vi "KRing Test.vi"() -> ()   [LabVIEW 2015]
uses:
  Controls/KRing/KRing.xctl
panel:
  out "Array":i16[](array[numeric])
  in  "Array":i16[](array[numeric])
  in  "KRing":i16(xcontrol)
  in  "Apply":bool
  in  "stop":bool
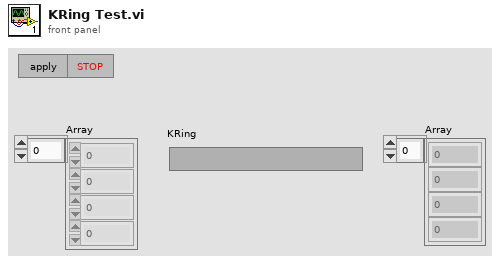
[diagram p1: front panel]
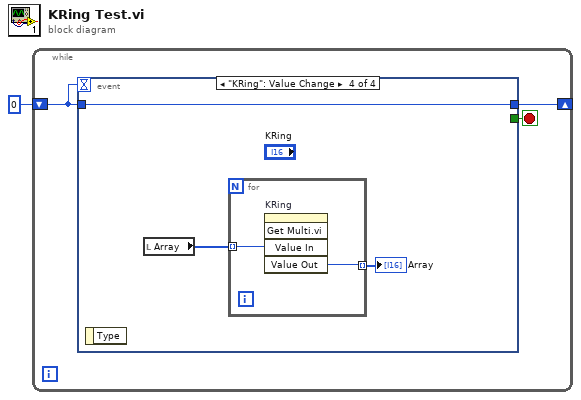
[diagram p0: block diagram]
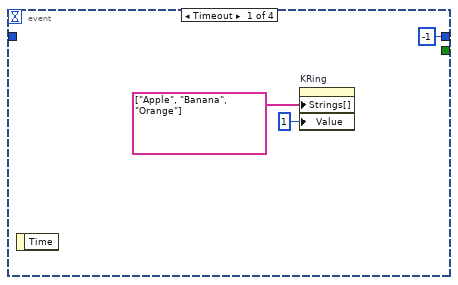
[diagram p2: hidden frame]
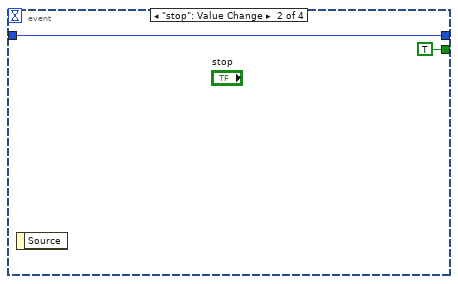
[diagram p3: hidden frame]
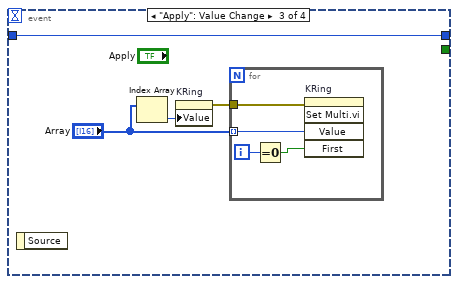
[diagram p4: hidden frame]
diagram:
  n1 = while {
    shift-right: [w2] -> _
    shift-left: 0 -> [w3]
    stop <- w4 stop-if-true
    n2 = event shown="[3] \"KRing\": Value Change" {
      selector: _ -> [_ _ _ _]
      dyn-events: _ -> [_ _ _ _]
      timeout: w3 -> [_ _ _ _]
      tunnel: [_ TRUE _ _] -> w4
      tunnel: w3 -> [_ w8 w13 w20]
      tunnel: [-1 w8 w13 w20] -> w2
      event Timeout {
        n3 = event-data() -> ()  [unwired: 1 in, 1 out]
        n4 = property on="KRing" class="KRing (strict)"("Strings[]"=string[] ["Apple", "Banana", "Orange"] ("Strings []"), "Value"=i16 1 ("KRing")) -> ()  [unwired: 2 in, 2 out]
      }
      event "stop": Value Change {
        n5 = event-data() -> ()  [unwired: 1 in, 1 out]
      }
      event "Apply": Value Change {
        n6 = event-data() -> ()  [unwired: 1 in, 1 out]
        n7 = Index Array(array="Array") -> (element=w10:i16)  [unwired: 1 in]
        n8 = property on="KRing" class="KRing (strict)"("Value"=w10) -> (error out=w12:errorcluster)  [unwired: 2 in, 1 out]
        n9 = for {
          tunnel: "Array" -> [w17] mode=indexing
          tunnel: w12 -> [w14]
          i -> [w16]
          n10 = Equal To 0?(x=w16) -> (x = 0?=w15:bool)
          n11 = invoke on="KRing" class="KRing (strict)" method="Set Multi.vi"(error in=w14, "Value"=w17, "First"=w15) -> ()  [unwired: 2 in, 5 out]
        }
      }
      event "KRing": Value Change {
        n12 = event-data() -> ()  [unwired: 1 in, 1 out]
        n13 = local read "Array"() -> (w19:i16[])
        n14 = for {
          tunnel: w19 -> [w22] mode=indexing
          tunnel: [w21] -> w18 mode=indexing
          n15 = invoke on="KRing" class="KRing (strict)" method="Get Multi.vi"("Value In"=w22) -> ("Value Out"=w21:i16)  [unwired: 4 in, 4 out]
        }
        "Array" <- w18
      }
    }
  }
